vi "Virtual Camera Start Stream.vi"(4 "Auto-Infuse":bool, 5 "Injection Countdown":bool, 6 "Shutter to Open":T1=enum."Cy3 (532 nm)", 7 "Auto Shutter":bool, 8 "error in (no error)":errorcluster, 9 "File Path":path, 10 "Camera Settings":T2={"Exposure Time (ms)"=100.0, "Binning"=enum."2x2", "Scan Mode (Flash)"=enum."Fast", "Trigger Mode (Flash)"=enum."Fast", "Frames to Acquire"=1000.0, "Pixel Correction (Flash)"=FALSE} {"Exposure Time (ms)" min=1.0 max=10000.0 step=1.0}, 11 "Virtual Camera in":refnum<class "Virtual Camera.lvclass">) -> (0 "error out":errorcluster, 3 "Virtual Camera out":refnum<class "Virtual Camera.lvclass">)   [LabVIEW 2018, in "Virtual Camera.lvlib" / "Virtual Camera.lvclass"]
uses:
  Virtual Camera.lvclass
  Resources/GLOBAL/GLOBAL Time-critical.vi
  Orca-Flash 4.0 V2 Messages/Flash Start Stream Msg/Flash Start Stream Msg.lvclass
  Synchronization Device/Synchronization Device.lvclass
  <vilib>/ActorFramework/Actor/Actor.lvclass
  Application Messages/Open Shutter Msg/Open Shutter Msg.lvclass
  User Interface/Countdown Timer/Countdown Timer.lvclass
  Application Messages/Pump Infuse Msg/Pump Infuse Msg.lvclass
  C:/Program Files/National Instruments/LabVIEW 2018/vi.lib/ActorFramework/Actor/Actor.lvclass
  Resources/Type Defs/Camera Settings.ctl
  Resources/Type Defs/Excitation.ctl
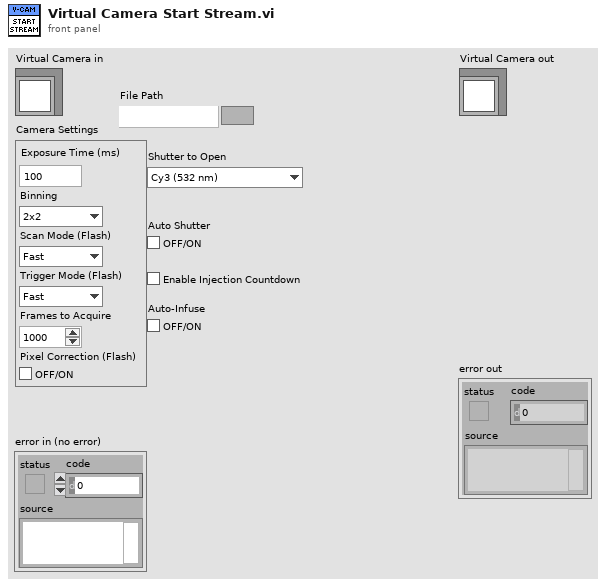
[diagram p1: front panel]
types:
  T1 = typedef "Excitation.ctl" = enum16{"Cy2 (473 nm)", "Cy3 (532 nm)", "Cy5 (639 nm)", "Cy7 (730 nm)", "Cy2/Cy3", "Cy3/Cy5", "Cy3/Cy7", "Cy5/Cy7"}
  T2 = typedef "Camera Settings.ctl" = cluster{"Exposure Time (ms)":dbl, "Binning":enum16{"1x1", "2x2", "4x4"}, "Scan Mode (Flash)":enum16{"Fast", "Slow"}, "Trigger Mode (Flash)":enum16{"Fast", "Standard"}, "Frames to Acquire":dbl, "Pixel Correction (Flash)":bool}
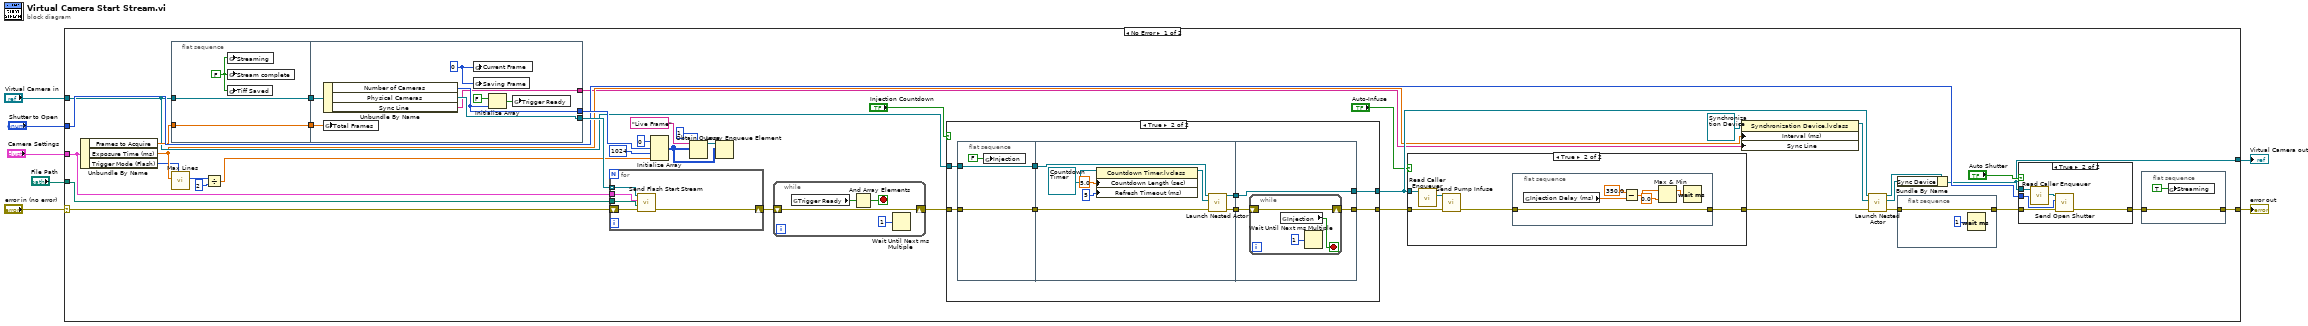
[diagram p0: block diagram]
diagram:
  n1 = case shown="No Error" "error in (no error)" {
    selector: "error in (no error)" -> [w40 w116]
    tunnel: [w33 w116] -> w6
    tunnel: [w31 w117] -> w4
    tunnel: "Virtual Camera in" -> [w23 w117]
    tunnel: "Camera Settings" -> [w42 _]
    tunnel: "File Path" -> [w43 _]
    tunnel: "Shutter to Open" -> [w36 _]
    frame No Error {
      n2 = Unbundle By Name(w42) -> ("Frames to Acquire"=w35:dbl, "Exposure Time (ms)"=w14:dbl, "Trigger Mode (Flash)"=w13:enum16{"Fast", "Standard"})
      n3 = flat-sequence {
        tunnel: w35 -> [w106]
        tunnel: w23 -> [w107]
        tunnel: [w107] -> w30
        tunnel: [w106] -> w29
        tunnel: [w115] -> w41
        tunnel: [w111] -> w44
        tunnel: w30 -> [w114]
        tunnel: w29 -> [w110]
        tunnel: [w108] -> w8
        frame #0 {
          w105 = FALSE ("Streaming")
          n4 = global write "GLOBAL Time-critical.vi" "Streaming"(w105) -> ()
          n5 = global write "GLOBAL Time-critical.vi" "Stream complete"(w105) -> ()
          n6 = global write "GLOBAL Time-critical.vi" "Tiff Saved"(w105) -> ()
        }
        frame #1 {
          w109 = 0 ("Current Frame")
          n7 = Unbundle By Name(w114) -> ("Number of Cameras"=w111:i32, "Physical Cameras"=w115:refnum<class "Message Enqueuer.lvclass">[], "Sync Line"=w108:tag)
          n8 = global write "GLOBAL Time-critical.vi" "Total Frames"(w110) -> ()
          n9 = global write "GLOBAL Time-critical.vi" "Current Frame"(w109) -> ()
          n10 = global write "GLOBAL Time-critical.vi" "Saving Frame"(w109) -> ()
          n11 = Initialize Array(FALSE, w111) -> (w112:bool[])
          n12 = global write "GLOBAL Time-critical.vi" "Trigger Ready"(w112) -> ()
        }
      }
      n13 = call "Max Lines.vi"("Trigger Mode"=w13, "Frame Time (ms)"=w14) -> ("Max Lines"=w28:i32)  [unwired: 8 in, 1 out]
      n14 = Divide(x=w28, y=2) -> (x/y=w26:dbl)
      n15 = for {
        tunnel: w43 -> [w98]
        tunnel: w42 -> [w97]
        tunnel: w41 -> [w96] mode=indexing
        shift-right: [w94] -> w39
        shift-left: w40 -> [w95]
        n16 = call "Send Flash Start Stream.vi"("error in (no error)"=w95, "File Path"=w98, "Camera Settings"=w97, "Message Enqueuer"=w96) -> ("error out"=w94:errorcluster)  [unwired: 6 in, 1 out]
      }
      n17 = Initialize Array(u16 0, w44, 1024 ("dimension size"), w26) -> (w9:u16[][][])
      n18 = Obtain Queue(max queue size (-1, unlimited)=1, name (unnamed)="Live Frame", element data type=w9) -> (queue out=w10:refnum<queue>)  [unwired: 2 in, 2 out]
      n19 = Lossy Enqueue Element(queue=w10, element=w9) -> ()  [unwired: 1 in, 4 out]
      n20 = while {
        shift-right: [w102] -> w22
        shift-left: w39 -> [w102]
        stop <- w100 stop-if-true
        n21 = global read "GLOBAL Time-critical.vi" "Trigger Ready"() -> (w101:bool[])
        n22 = And Array Elements(Boolean array=w101) -> (logical AND=w100:bool)
        n23 = Wait Until Next ms Multiple(millisecond multiple=u32 1) -> ()  [unwired: 1 out]
      }
      n24 = case shown="True" "Injection Countdown" {
        tunnel: w23 -> [w62 w70]
        tunnel: [w62 w69] -> w16
        tunnel: w22 -> [w61 w68]
        tunnel: [w61 w65] -> w18
        frame False {
        }
        frame True {
          n25 = flat-sequence {
            tunnel: w68 -> [w72]
            tunnel: w70 -> [w73]
            tunnel: [w73] -> w67
            tunnel: [w72] -> w66
            tunnel: w67 -> [w81]
            tunnel: w66 -> [w75]
            tunnel: [w80] -> w64
            tunnel: [w74] -> w63
            tunnel: [w82] -> w65
            tunnel: [w84] -> w69
            tunnel: w64 -> [w84]
            tunnel: w63 -> [w83]
            frame #0 {
              n26 = global write "GLOBAL Time-critical.vi" "Injection"(FALSE ("Injection")) -> ()
            }
            frame #1 {
              n27 = property class="Countdown Timer.lvclass"(reference=refnum<class "Countdown Timer.lvclass"> refnum ("Countdown Timer.lvlib:Countdown Timer.lvclass"), "Countdown Length (sec)"=5.0, "Refresh Timeout (ms)"=5) -> (reference out=w76:refnum<class "Countdown Timer.lvclass">)  [unwired: 1 in, 1 out]
              n28 = call <vilib>:"Launch Nested Actor.vi"("error in (no error)"=w75, "Nested Actor"=w76, "Caller Actor in"=w81) -> ("error out"=w74:errorcluster, "Caller Actor out"=w80:refnum<class "Virtual Camera.lvclass">)  [unwired: 6 in, 1 out]
            }
            frame #2 {
              n29 = while {
                shift-right: [w87] -> w82
                shift-left: w83 -> [w87]
                stop <- w85 stop-if-true
                n30 = global read "GLOBAL Time-critical.vi" "Injection"() -> (w85:bool)
                n31 = Wait Until Next ms Multiple(millisecond multiple=u32 1) -> ()  [unwired: 1 out]
              }
            }
          }
        }
      }
      n32 = case shown="True" "Auto-Infuse" {
        tunnel: w16 -> [_ w52]
        tunnel: w18 -> [w47 w50]
        tunnel: [w47 w48] -> w17
        frame False {
        }
        frame True {
          n33 = call <vilib>:"Read Caller Enqueuer.vi"("Actor"=w52) -> ("Caller Enqueuer"=w51:refnum<class "Message Enqueuer.lvclass">)  [unwired: 10 in]
          n34 = call "Send Pump Infuse.vi"("error in (no error)"=w50, "Message Enqueuer"=w51) -> ("error out"=w49:errorcluster)  [unwired: 8 in, 1 out]
          n35 = flat-sequence {
            tunnel: w49 -> [w58]
            tunnel: [w58] -> w48
            frame #0 {
              n36 = global read "GLOBAL Time-critical.vi" "Injection Delay (ms)"() -> (w56:dbl)
              n37 = Subtract(x=350.0, y=w56) -> (x-y=w55:dbl)
              n38 = Max & Min(x=w55, y=0.0) -> (max(x,y)=w53:dbl)  [unwired: 1 out]
              n39 = Wait (ms)(milliseconds to wait=w53) -> ()  [unwired: 1 out]
            }
          }
        }
      }
      n40 = property class="Synchronization Device.lvclass"(reference=refnum<class "Synchronization Device.lvclass"> refnum ("Synchronization Device.lvlib:Synchronization Device.lvclass"), "Interval (ms)"=w14, "Sync Line"=w8) -> (reference out=w37:refnum<class "Synchronization Device.lvclass">)  [unwired: 1 in, 1 out]
      n41 = call <vilib>:"Launch Nested Actor.vi"("error in (no error)"=w17, "Nested Actor"=w37, "Caller Actor in"=w16) -> ("error out"=w20:errorcluster, "Nested Actor's Enqueuer"=w25:refnum<class "Message Enqueuer.lvclass">, "Caller Actor out"=w24:refnum<class "Virtual Camera.lvclass">)  [unwired: 6 in]
      n42 = Bundle By Name(cluster=w24, "Sync Device"=w25) -> (w31:refnum<class "Virtual Camera.lvclass">)
      n43 = flat-sequence {
        tunnel: w20 -> [w60]
        tunnel: [w60] -> w19
        frame #0 {
          n44 = Wait (ms)(milliseconds to wait=u32 1) -> ()  [unwired: 1 out]
        }
      }
      n45 = case shown="True" "Auto Shutter" {
        tunnel: w36 -> [_ w93]
        tunnel: w19 -> [w88 w92]
        tunnel: [w88 w91] -> w34
        tunnel: w31 -> [_ w90]
        frame False {
        }
        frame True {
          n46 = call <vilib>:"Read Caller Enqueuer.vi"("Actor"=w90) -> ("Caller Enqueuer"=w89:refnum<class "Message Enqueuer.lvclass">)  [unwired: 10 in]
          n47 = call "Send Open Shutter.vi"("error in (no error)"=w92, "Shutter to Open"=w93, "Message Enqueuer"=w89) -> ("error out"=w91:errorcluster)  [unwired: 7 in, 1 out]
        }
      }
      n48 = flat-sequence {
        tunnel: w34 -> [w103]
        tunnel: [w103] -> w33
        frame #0 {
          n49 = global write "GLOBAL Time-critical.vi" "Streaming"(TRUE ("Streaming")) -> ()
        }
      }
    }
    frame Error {
    }
  }
  "error out" <- w6
  "Virtual Camera out" <- w4
